vi "Write Color.vi"(8 "error in (no error)":errorcluster, 10 "Color in":u32(colorbox), 11 "CircleShape in":refnum<class "CircleShape.lvclass">) -> (0 "error out":errorcluster, 3 "CircleShape out":refnum<class "CircleShape.lvclass">)   [LabVIEW 2022 SP3, in "CircleShape.lvclass"]
uses:
  CircleShape.lvclass
  CircleShape.lvclass/CircleShape.ctl
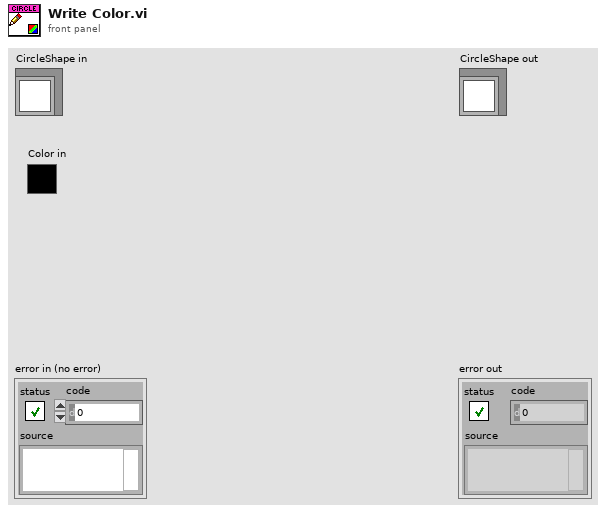
[diagram p1: front panel]
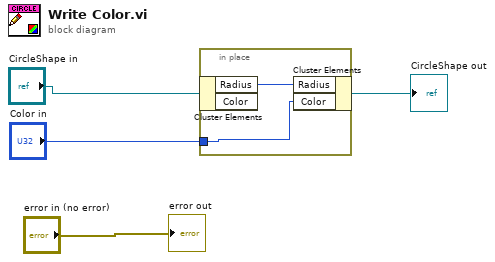
[diagram p0: block diagram]
diagram:
  n1 = in-place {
    in-place-border: "Color in" -> [w5]
    n2 = in-place-cluster #1("CircleShape in") -> ("Radius"=w6:i16)  [unwired: 1 out]
    n3 = in-place-cluster #1("Radius"=w6, "Color"=w5) -> (→"CircleShape out":refnum<class "CircleShape.lvclass">)
  }
  "error out" <- "error in (no error)"
